vi "Write Splitters.vi"(8 "error in":errorcluster, 10 "Splitters":refnum<vi>[](array[refnum]), 11 "Base Software in":refnum<class "Main.lvclass">) -> (0 "error out":errorcluster, 3 "Base Software out":refnum<class "Main.lvclass">)   [LabVIEW 2023, in "Main.lvlib" / "Main.lvclass"]
doc: "Array of splitter references in Order Shall be:\n0 Top\n1 Right\n2 Bottom \n3 Left"
uses:
  Project/Main.lvclass
  Project/Main.lvclass/Main.ctl
  builds/Engine/Engine.lvlibp/Project/Engine.lvclass
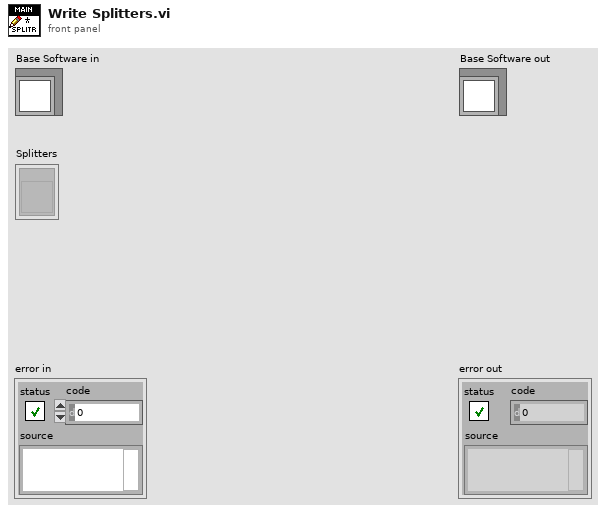
[diagram p1: front panel]
types:
  T1 = typedef "Main.lvlib/Main.lvclass/Splitters.ctl" = cluster{"Splitter":refnum<vi>, "Initial":i32}
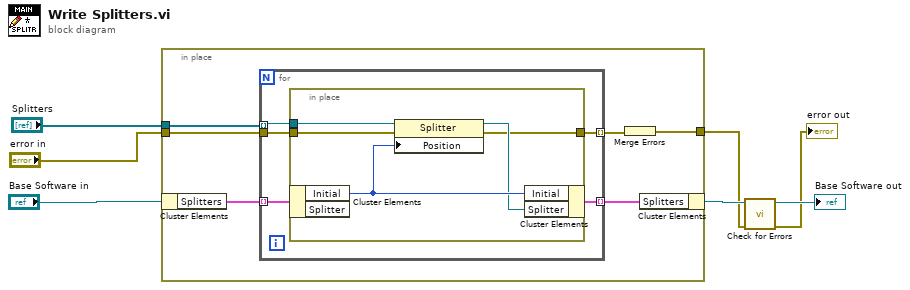
[diagram p0: block diagram]
diagram:
  n1 = in-place {
    in-place-border: "Splitters" -> [w12]
    in-place-border: "error in" -> [w10]
    in-place-border: [w8] -> w2
    n2 = in-place-cluster #1("Base Software in") -> ("Splitters"=w13:T1[])
    n3 = for {
      tunnel: w13 -> [w17] mode=indexing
      tunnel: w12 -> [w18] mode=indexing
      tunnel: [w16] -> w11 mode=indexing
      tunnel: w10 -> [w15]
      tunnel: [w14] -> w9 mode=indexing
      n4 = in-place {
        in-place-border: w18 -> [w23]
        in-place-border: w15 -> [w20]
        in-place-border: [w19] -> w14
        n5 = in-place-cluster #2(w17) -> ("Initial"=w22:i32)  [unwired: 1 out]
        n6 = property class="Splitter"(reference=w23, error in=w20, "Position"=w22) -> (reference out=w21:refnum<vi>, error out=w19:errorcluster)
        n7 = in-place-cluster #2("Initial"=w22, "Splitter"=w21) -> (w16:T1)
      }
    }
    n8 = Merge Errors(w9) -> (w8:errorcluster)
    n9 = in-place-cluster #1("Splitters"=w11) -> (w4:refnum<class "Main.lvclass">)
  }
  n10 = call "Check for Errors.vi"("error in"=w2, "Engine in"=w4) -> ("error out"=→"error out":errorcluster, "Engine out"=→"Base Software out":refnum<class "Main.lvclass">)  [unwired: 8 in]
